vi "Index.vi"(8 "error in (no error)":errorcluster, 10 "Index":i32, 11 "I32 Array in":refnum<class "I32 Array.lvclass">) -> (0 "error out":errorcluster, 3 "Indexed element":refnum<class "Generic Data.lvclass">)   [LabVIEW 2020, in "Data.lvlib" / "I32 Array.lvclass"]
doc: "Index an element from 'Generic Data in'.\nThis implementation returns a generic U32 class with the indexed U32."
uses:
  I32 Array.lvclass
  Generic Data.lvclass
  I32 Array.lvclass/I32 Array.ctl
  I32/I32.lvclass/I32.ctl
  I32/I32.lvclass
  C:/Users/Henri/OneDrive/LabVIEW/Framework/Data/Generic Data/Generic Data.lvclass
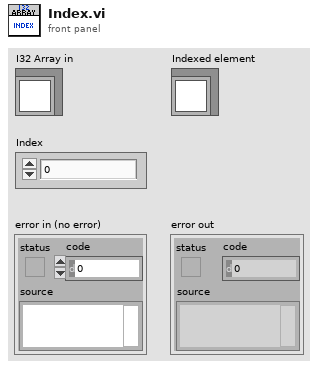
[diagram p1: front panel]
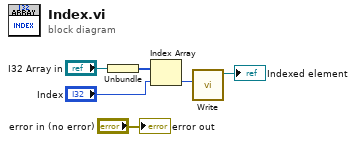
[diagram p0: block diagram]
diagram:
  n1 = Unbundle("I32 Array in") -> (w5:i32[])
  n2 = Index Array(array=w5, index="Index") -> (element=w2:i32)
  n3 = call "Write.vi"("I32"=w2) -> ("I32 out"=→"Indexed element":refnum<class "I32.lvclass">)  [unwired: 10 in]
  "error out" <- "error in (no error)"
